vi "Write Path.vi"(8 "error in (no error)":errorcluster, 9 "Experiment name":string, 10 "Path":path=path "C:/Users/YuanYuan/Desktop/Labview Data/Chirp", 11 "ChirpEIS In":refnum<class "ChirpEIS.lvclass">) -> (0 "error out":errorcluster, 3 "ChirpEIS out":refnum<class "ChirpEIS.lvclass">)   [LabVIEW 2014, in "ChirpEIS.lvclass"]
uses:
  ChirpEIS.lvclass
  ChirpEIS.lvclass/ChirpEIS.ctl
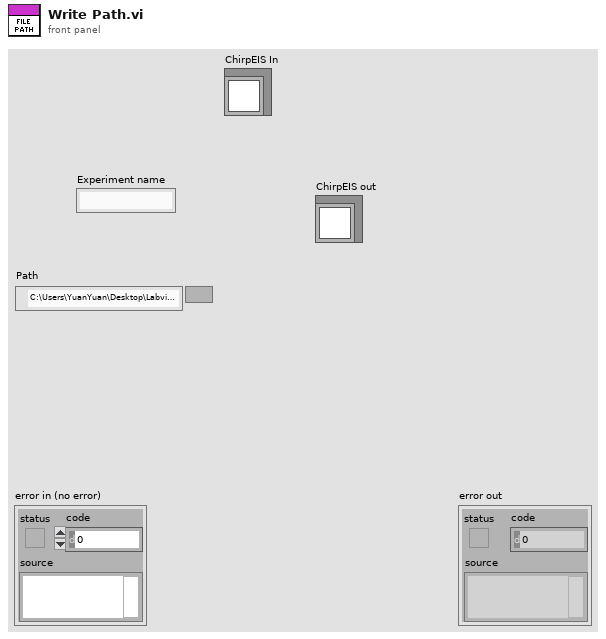
[diagram p1: front panel]
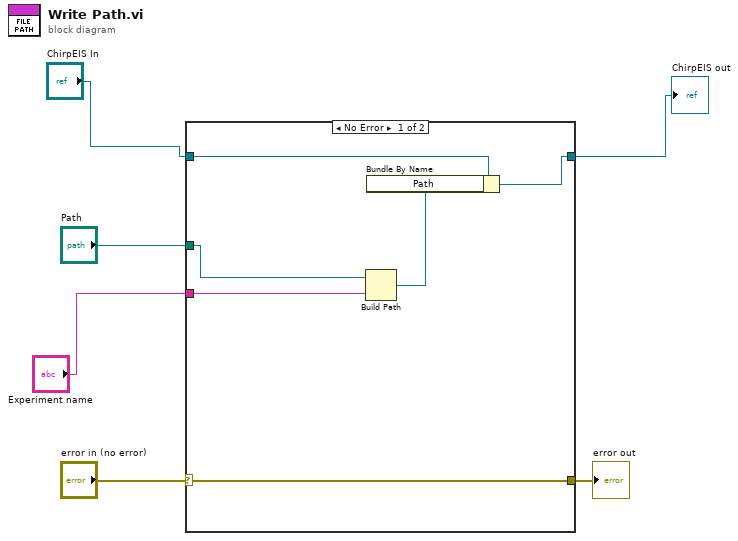
[diagram p0: block diagram]
diagram:
  n1 = case shown="No Error" "error in (no error)" {
    selector: "error in (no error)" -> [w12 w13]
    tunnel: [w12 w13] -> w5
    tunnel: [w7 w14] -> w2
    tunnel: "ChirpEIS In" -> [w9 w14]
    tunnel: "Path" -> [w11 _]
    tunnel: "Experiment name" -> [w10 _]
    frame No Error {
      n2 = Build Path(base path=w11, name or relative path=w10) -> (appended path=w8:path)
      n3 = Bundle By Name(cluster=w9, "Path"=w8) -> (w7:refnum<class "ChirpEIS.lvclass">)
    }
    frame Error {
    }
  }
  "error out" <- w5
  "ChirpEIS out" <- w2
